vi "Move XZ Raster.vi"(4 "Initial Z Direction":bool=TRUE, 6 "Initial X Direction":bool=TRUE, 8 "Error In":errorcluster, 9 "Z Number of Steps":string="0", 10 "X Number of Steps":string="0", 11 "Reference In":refnum<class "_Controller.lvclass">) -> (0 "Error Out":errorcluster, 3 "Reference Out":refnum<class "_Controller.lvclass">)   [LabVIEW 2020]
doc: "Bi-axial raster scan logic for the XZ plane. Performs the uni-axial raster scan logic in the X direction then moves along 1 scanning point in the Z dirction. This is the looped to cover the entire area.\n\nArgs:\n\nReference In: Incoming communication (reference) between LabView and the scanning rig controller\nX Number of Steps: Total number of steps to move along that axis\nZ Number of Steps: Total number of steps to move along that axis\nInitial X Direction: Initial X direction for the scan\nInitial Z Direction: Initial Z direction for the scan\nError In: Checks for any errors with the incoming communication (reference)\n\nReturns:\n\nReference Out: Output communnication (reference) between LabView and controller\nError Out: Checks for any error with output communication (reference)"
uses:
  <instrlib>/Arcus Ethernet Driver 1.0.0/ArcusEthernetComm/classes/Controller/_Controller.lvclass
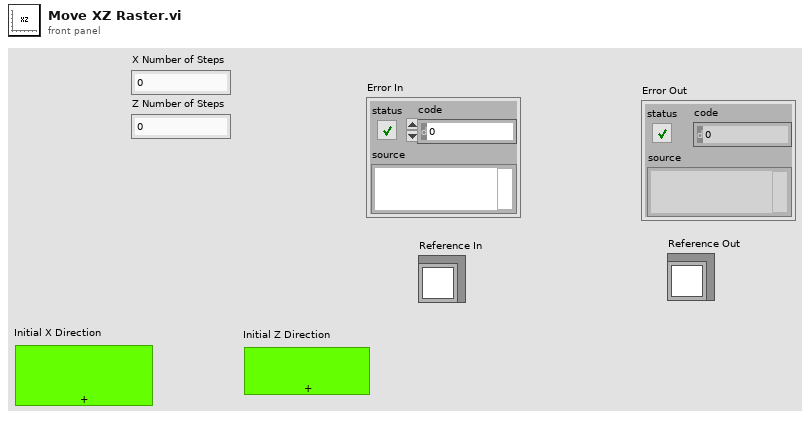
[diagram p1: front panel]
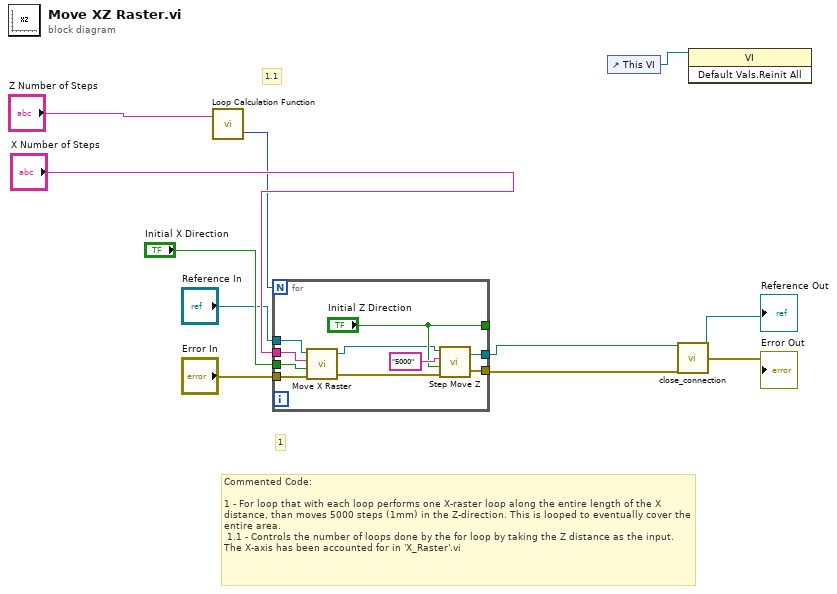
[diagram p0: block diagram]
diagram:
  # "Commented Code:\n\n1 - For loop that with each loop performs one X-raster loop along the entire length of the X distance, than moves 5000 steps (1mm) in the Z-direction. This is looped to eventually cover the entire area.\n 1.1 - Controls the number of loops done by the for loop by taking the Z distance as the input. The X-axis has been accounted for in 'X_Raster'.vi"
  # "1.1"
  # "1"
  n1 = call "Loop Calculation Function.vi"("Number of Steps"="Z Number of Steps") -> ("No. of Scan Points"=w5:i32)  [unwired: 1 in, 1 out]
  n2 = for {
    N: w5 -> [_]
    tunnel: "X Number of Steps" -> [w19]
    tunnel: "Initial X Direction" -> [w20]
    tunnel: ["Initial Z Direction"] -> _
    tunnel: [w16] -> w2
    tunnel: [w15] -> w1
    tunnel: "Reference In" -> [w13]
    tunnel: "Error In" -> [w12]
    n3 = call "Move X Raster.vi"("Error In"=w12, "Initial Direction"=w20, "X Number of Steps"=w19, "Reference In"=w13) -> ("Error Out"=w14:errorcluster, "Reference Out"=w17:refnum<class "_Controller.lvclass">)  [unwired: 1 in]
    n4 = call "Step Move Z.vi"("Error In"=w14, "Direction"="Initial Z Direction", "No. of Z Steps"="5000" ("Y Steps"), "Reference In"=w17) -> ("Error Out"=w15:errorcluster, "Reference Out"=w16:refnum<class "_Controller.lvclass">)
  }
  n5 = control-ref of="This VI"() -> (w4:refnum<vi>)
  n6 = call <instrlib>:"close_connection.vi"("reference (in)"=w2, "error in (no error)"=w1) -> ("reference (out)"=→"Reference Out":refnum<class "_Controller.lvclass">, "error out"=→"Error Out":errorcluster)  [unwired: 16 in]
  n7 = invoke class="VI" method="Default Vals.Reinit All"(reference=w4) -> ()  [unwired: 2 in, 3 out]
